vi "IMAQ-Init.vi"(1 "Image Name":string) -> (0 "Image Device IN":cluster{"Image":T1, "errorImage":errorcluster})   [LabVIEW 2010]
uses:
  <vilib>/vision/Image Controls.llb/IMAQ Image.ctl
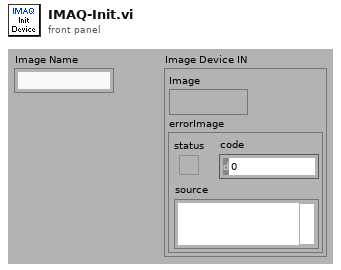
[diagram p1: front panel]
types:
  T1 = typedef "IMAQ Image.ctl" = refnum<image>
  T2 = typedef "Image Type" = u32
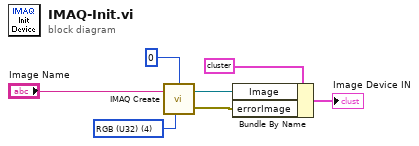
[diagram p0: block diagram]
diagram:
  w3 = T2 4 items=["Grayscale (U8)", "Grayscale (I16)", "Grayscale (SGL)", "Complex (CSG)", "RGB (U32)", "HSL (U32)", "RGB (U64)", "Grayscale (U16)"] ("Image Type")
  n1 = call "IMAQ Create"("Border Size"=0, "Image Name"="Image Name", "Image Type"=w3) -> ("New Image"=w2:T1, "error out"=w1:errorcluster)  [unwired: 2 in]
  n2 = Bundle By Name(cluster=cluster{"Image":T1, "errorImage":errorcluster} {"Image"=refnum, "errorImage"={"status"=FALSE, "code"=0, "source"=""}} ("Image Device IN"), "Image"=w2, "errorImage"=w1) -> (→"Image Device IN":cluster{"Image":T1, "errorImage":errorcluster})
